vi "Instruction for User.vi"(8 "End-point entered?":bool, 11 "GO?":bool) -> (1 "User Instruction":T1(ring))   [LabVIEW 2016]
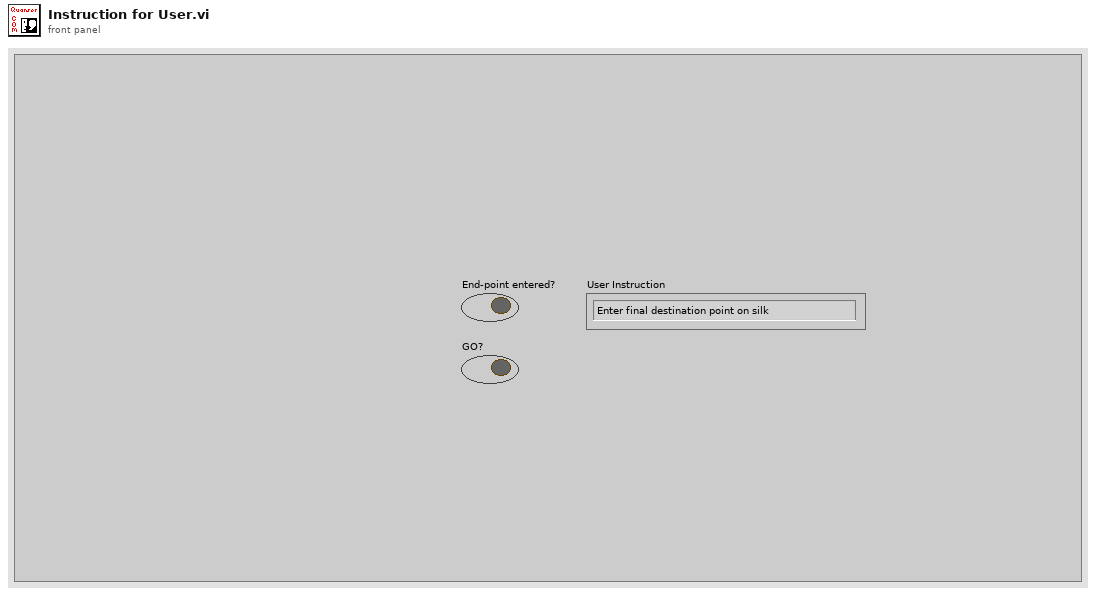
[diagram p1: front panel]
types:
  T1 = enum16{"Enter final destination point on silk", "Enter way-points if any, and hit GO! when ready", "Look at it go!"}
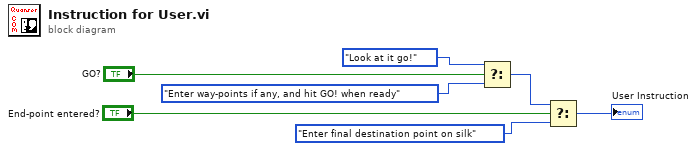
[diagram p0: block diagram]
diagram:
  n1 = Select(t=T1."Look at it go!", s="GO?", f=T1."Enter way-points if any, and hit GO! when ready") -> (s? t:f=w6:T1)
  n2 = Select(t=w6, s="End-point entered?", f=T1."Enter final destination point on silk") -> (s? t:f=→"User Instruction":T1)
